vi "ZoomAndSlide.vi"(0 "Scene.Object IN":refnum<vi>, 1 "Final Position":sgl, 2 "Final Zoom":sgl, 3 "Resolution":i32=50) -> (5 "Scene.Object Out":refnum<vi>)   [LabVIEW 2010]
uses:
  chrisbuerginrogers/Documents/RoboSlides/RoboSlides1b5.llb/SlideGlobals.vi
  <vilib>/picture/3D Picture Control/NI_3D Picture Control.lvlib
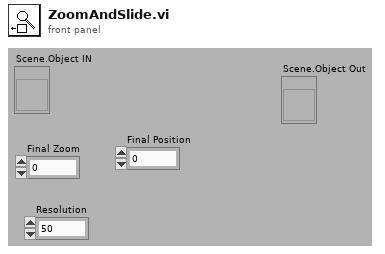
[diagram p1: front panel]
types:
  T1 = typedef "LV3DPointTypeDef.ctl" = cluster{"X":sgl, "Y":sgl, "Z":sgl}
  T2 = cluster{"Final Zoom":sgl, "Final Zoom":sgl, "Final Zoom":sgl}
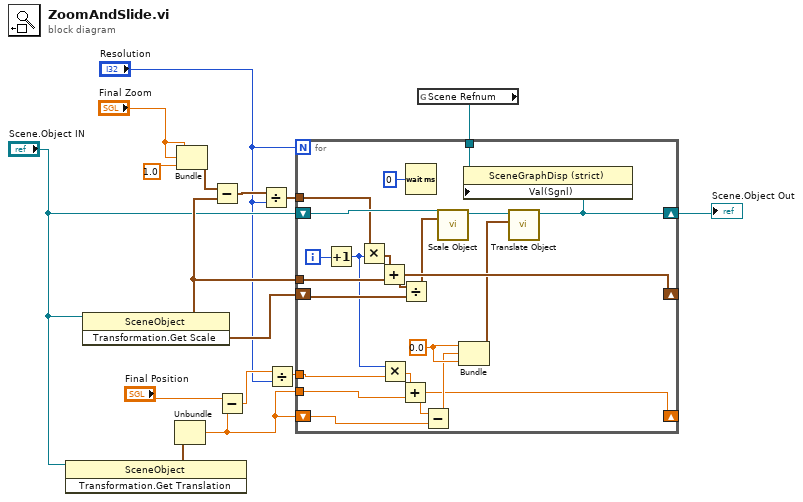
[diagram p0: block diagram]
diagram:
  n1 = invoke class="SceneObject" method="Transformation.Get Translation"(reference="Scene.Object IN") -> ("Transformation.GetTranslation"=w6:T1)  [unwired: 2 in, 2 out]
  n2 = invoke class="SceneObject" method="Transformation.Get Scale"(reference="Scene.Object IN") -> ("Transformation.Get Scale"=w14:T1)  [unwired: 2 in, 2 out]
  n3 = Unbundle(w6) -> ("Y"=w2:sgl)  [unwired: 2 out]
  n4 = Bundle("Final Zoom"="Final Zoom", "Final Zoom"="Final Zoom", "Final Zoom"=sgl 1.0) -> (w11:T2)  [unwired: 1 in]
  n5 = Subtract(x=w11, y=w14) -> (x-y=w12:T1)
  n6 = Subtract(x="Final Position", y=w2) -> (x-y=w7:sgl)
  n7 = Divide(x=w12, y="Resolution") -> (x/y=w13:T1)
  n8 = Divide(x=w7, y="Resolution") -> (x/y=w3:sgl)
  n9 = global read "SlideGlobals.vi" "Scene Refnum"() -> (w1:refnum<vi>)
  n10 = for {
    N: "Resolution" -> [_]
    shift-right: [w16] -> w15
    shift-left: "Scene.Object IN" -> [w34]
    tunnel: w13 -> [w33]
    tunnel: w14 -> [w35]
    shift-right: [w31] -> _
    shift-left: w14 -> [w32]
    tunnel: w1 -> [w29]
    shift-right: [w23] -> _
    shift-left: w2 -> [w22]
    tunnel: w3 -> [w20]
    tunnel: w2 -> [w19]
    i -> [w24]
    w27 = sgl 0.0 ("Final Zoom")
    n11 = Increment(x=w24) -> (x+1=w21:i32)
    n12 = Multiply(x=w33, y=w21) -> (x*y=w36:T1)
    n13 = Add(x=w36, y=w35) -> (x+y=w31:T1)
    n14 = Multiply(x=w21, y=w20) -> (x*y=w28:sgl)
    n15 = Add(x=w28, y=w19) -> (x+y=w23:sgl)
    n16 = Divide(x=w31, y=w32) -> (x/y=w30:T1)
    n17 = Wait (ms)(milliseconds to wait=u32 0) -> ()  [unwired: 1 out]
    n18 = Subtract(x=w23, y=w22) -> (x-y=w25:sgl)
    n19 = call <vilib>:"Scale Object.vi"("Scale"=w30, "Scene.Object In"=w34) -> ("Scene.Object Out"=w17:refnum<vi>)  [unwired: 8 in, 1 out]
    n20 = Bundle("Final Zoom"=w27, w25, "Final Zoom"=w27) -> (w26:cluster{"Final Zoom":sgl, sgl, "Final Zoom":sgl})  [unwired: 1 in]
    n21 = call <vilib>:"Translate Object.vi"("Translation"=w26, "Scene.Object In"=w17) -> ("Scene.Object Out"=w16:refnum<vi>)  [unwired: 8 in, 1 out]
    n22 = property class="SceneGraphDisp (strict)"(reference=w29, "Val(Sgnl)"=w16) -> ()  [unwired: 1 in, 2 out]
  }
  "Scene.Object Out" <- w15
